vi "RellenarMatriz.vi"() -> ()   [LabVIEW 2022 SP3]
panel:
  out "Matriz":dbl[][](array[numeric])
  # "Arrays en LabVIEW"
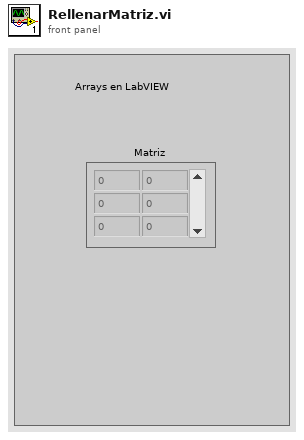
[diagram p1: front panel]
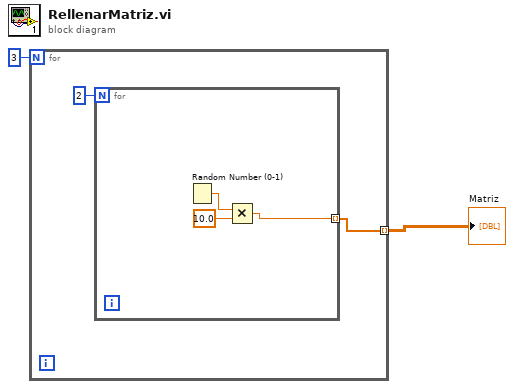
[diagram p0: block diagram]
diagram:
  n1 = for {
    N: 3 -> [_]
    tunnel: [w3] -> w1 mode=indexing
    n2 = for {
      N: 2 -> [_]
      tunnel: [w5] -> w3 mode=indexing
      n3 = Random Number (0-1)() -> (number: 0 to 1=w7:dbl)
      n4 = Multiply(x=w7, y=10.0) -> (x*y=w5:dbl)
    }
  }
  "Matriz" <- w1
